vi "Find Peak and Onset.vi"(5 "Static onset threshold (20 deg/s)":dbl=20.0 format="%#_13g", 7 "Use % Onset Threshold? (F)":bool, 8 "error in (no error)":errorcluster, 10 "Stimulus in":dbl[][](array[numeric]), 11 "Head Impulse Fit in":refnum<class "Head Impulse Fit.lvclass">) -> (0 "error out":errorcluster, 1 "Onset Indicies":i32[](array[numeric]), 2 "Peak Indicies":i32[](array[numeric]), 3 "Head Impulse Fit out":refnum<class "Head Impulse Fit.lvclass">)   [LabVIEW 2016, in "Head Impulse Fit.lvclass"]
uses:
  Head Impulse Fit.lvclass
  Head Impulse Fit.lvclass/Head Impulse Fit.ctl
  comm/stats/stats.lvlib
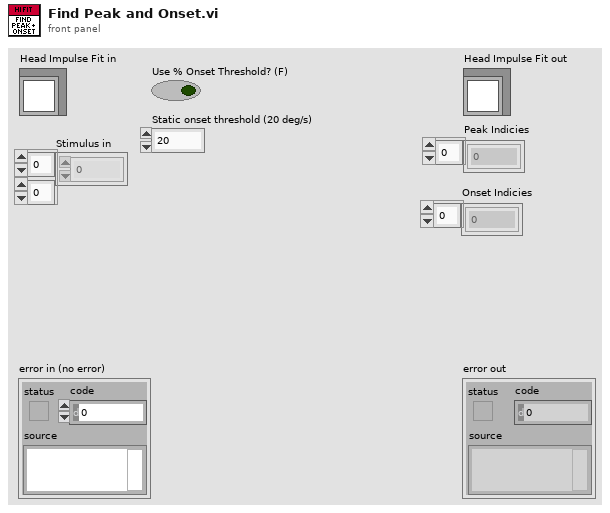
[diagram p1: front panel]
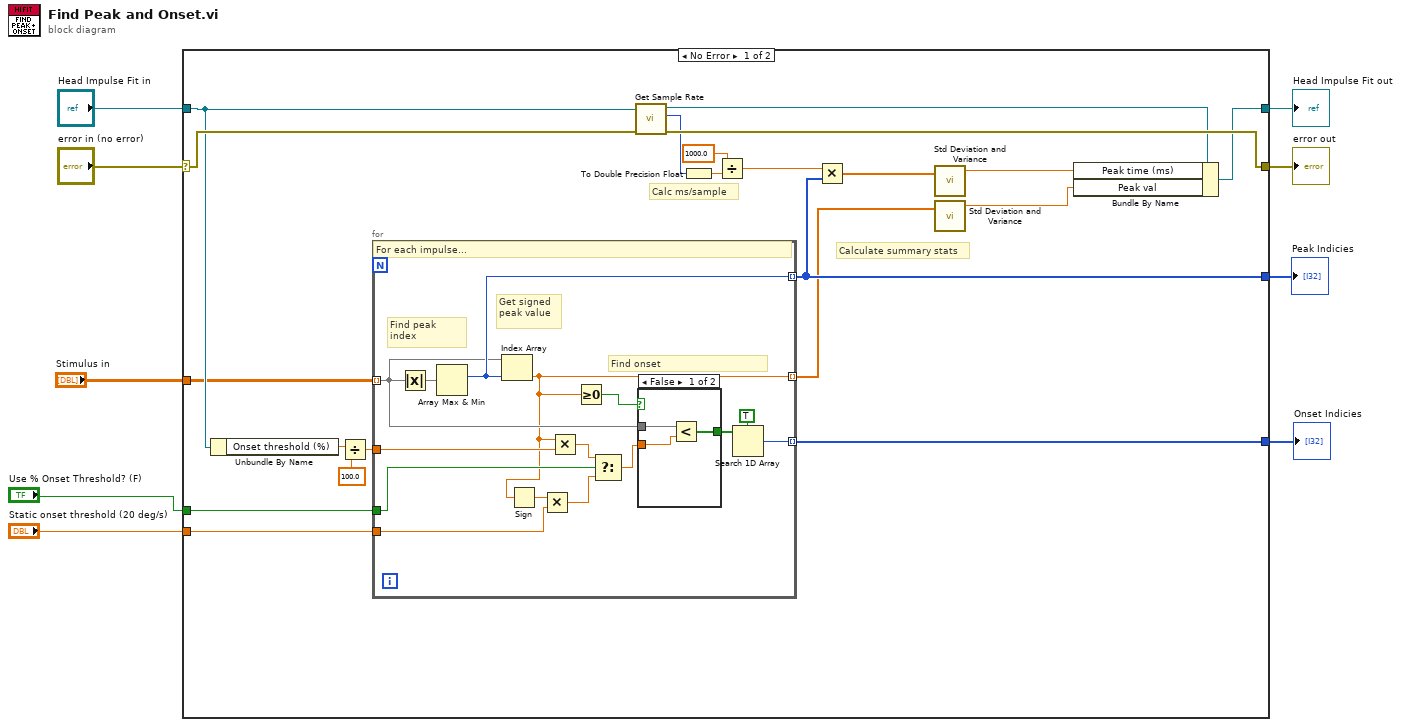
[diagram p0: block diagram]
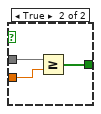
[diagram p2: hidden frame]
diagram:
  n1 = case shown="No Error" "error in (no error)" {
    selector: "error in (no error)" -> [w29 w53]
    tunnel: [w30 w53] -> w8
    tunnel: [w14 w52] -> w6
    tunnel: "Head Impulse Fit in" -> [w28 w52]
    tunnel: "Stimulus in" -> [w26 _]
    tunnel: [w22 _] -> w3
    tunnel: [w19 _] -> w4
    tunnel: "Use % Onset Threshold? (F)" -> [w11 _]
    tunnel: "Static onset threshold (20 deg/s)" -> [w10 _]
    frame No Error {
      # "Calculate summary stats"
      # "Calc ms/sample"
      n2 = Unbundle By Name(w28) -> ("Onset threshold (%)"=w25:dbl)
      n3 = Divide(x=w25, y=100.0) -> (x/y=w23:dbl)
      n4 = for {
        tunnel: [w34] -> w16 mode=indexing
        tunnel: [w40] -> w19 mode=indexing
        tunnel: w26 -> [w39] mode=indexing
        tunnel: w23 -> [w45]
        tunnel: [w41] -> w22 mode=indexing
        tunnel: w11 -> [w35]
        tunnel: w10 -> [w32]
        # "Get signed peak value"
        # "Find onset"
        # "Find peak\nindex"
        # "For each impulse..."
        n5 = Absolute Value(x=w39) -> (abs(x)=w44:dbl[])
        n6 = Array Max & Min(array=w44) -> (max index (indices)=w40:i32)  [unwired: 3 out]
        n7 = Index Array(array=w39, index=w40) -> (element=w34:dbl)
        n8 = Sign(1:w34) -> (0:w33:dbl)
        n9 = Multiply(x=w33, y=w32) -> (x*y=w31:dbl)
        n10 = Multiply(x=w34, y=w45) -> (x*y=w36:dbl)
        n11 = Greater Or Equal To 0?(x=w34) -> (x >= 0?=w38:bool)
        n12 = Select(t=w36, s=w35, f=w31) -> (s? t:f=w37:dbl)
        n13 = case shown="False" w38 {
          tunnel: [w46 w51] -> w43
          tunnel: w39 -> [w48 w50]
          tunnel: w37 -> [w47 w49]
          frame False {
            n14 = Less?(x=w48, y=w47) -> (x < y?=w46:bool[])
          }
          frame True {
            n15 = Greater Or Equal?(x=w50, y=w49) -> (x >= y?=w51:bool[])
          }
        }
        n16 = Search 1D Array(1D array=w43, element=TRUE) -> (index of element=w41:i32)  [unwired: 1 in]
      }
      n17 = call-dynamic "Get Sample Rate.vi"("error in (no error)"=w29, "Abstract Fit in"=w28) -> ("error out"=w30:errorcluster, "Sample Rate"=w27:i32, "Abstract Fit out"=w15:refnum<class "Head Impulse Fit.lvclass">)  [unwired: 7 in]
      n18 = To Double Precision Float(number=w27) -> (double precision float=w21:dbl)
      n19 = Divide(x=1000.0, y=w21) -> (x/y=w18:dbl)
      n20 = Multiply(x=w18, y=w19) -> (x*y=w17:dbl[])
      n21 = call "Std Deviation and Variance.vi"("X"=w17) -> ("mean"=w13:dbl)  [unwired: 1 in, 2 out]
      n22 = call "Std Deviation and Variance.vi"("X"=w16) -> ("mean"=w12:dbl)  [unwired: 1 in, 2 out]
      n23 = Bundle By Name(cluster=w15, "Peak time (ms)"=w13, "Peak val"=w12) -> (w14:refnum<class "Head Impulse Fit.lvclass">)
    }
    frame Error {
    }
  }
  "error out" <- w8
  "Head Impulse Fit out" <- w6
  "Peak Indicies" <- w4
  "Onset Indicies" <- w3
